vi "Check Valid.vi"(11 "IResult.lvclass":refnum<class "IResult2.lvclass">) -> (3 "Valid?":bool)   [LabVIEW 2020, in "IResult2.lvclass"]
uses:
  IResult2.lvclass
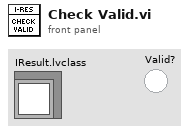
[diagram p1: front panel]
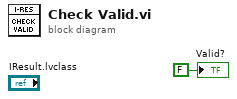
[diagram p0: block diagram]
diagram:
  "Valid?" <- FALSE ("Valid?")
